vi "Video Toolset Snapshot.vi"   [LabVIEW 2010]
uses:
  Video Toolset/vi/subvi/Remote Snapshot.vi
types:
  T1 = enum32{"Bad", "Idle", "Run top level", "Running"}
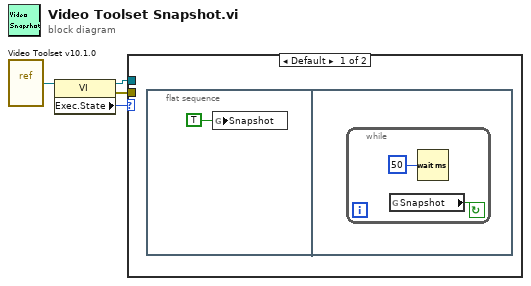
[diagram p0: block diagram]
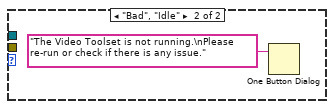
[diagram p2: hidden frame]
diagram:
  n1 = vi-ref "Video Toolset v10.1.0.vi"() -> (w4:refnum<vi>)
  n2 = property class="VI"(reference=w4) -> (reference out=w3:refnum<vi>, error out=w1:errorcluster, "Exec.State"=w2:T1)  [unwired: 1 in]
  n3 = case shown="Default" w2 {
    tunnel: w3 -> [_ _]
    tunnel: w1 -> [_ _]
    frame Default {
      n4 = flat-sequence {
        frame #0 {
          n5 = global write "Remote Snapshot.vi" "Snapshot"(TRUE ("Snapshot")) -> ()
        }
        frame #1 {
          n6 = while {
            stop <- w7 continue-if-true
            n7 = global read "Remote Snapshot.vi" "Snapshot"() -> (w7:bool)
            n8 = Wait (ms)(milliseconds to wait=u32 50) -> ()  [unwired: 1 out]
          }
        }
      }
    }
    frame "Bad", "Idle" {
      n9 = One Button Dialog(message="The Video Toolset is not running.\nPlease re-run or check if there is any issue.") -> ()  [unwired: 1 in, 1 out]
    }
  }
